vi "Lab2_Light_Filter.vi"() -> ()   [LabVIEW 2022 SP3]
uses:
  <vilib>/DAQmx/read.llb/DAQmx Read (Analog DBL 1Chan 1Samp).vi
  <vilib>/DAQmx/miscellaneous.llb/DAQmx Fill In Error Info.vi
panel:
  in  "stop":bool
  in  "L (0..1)":dbl
  out "error constant":errorcluster
  out "Waveform Chart":cluster{"data":dbl, "y2":dbl}(graph)
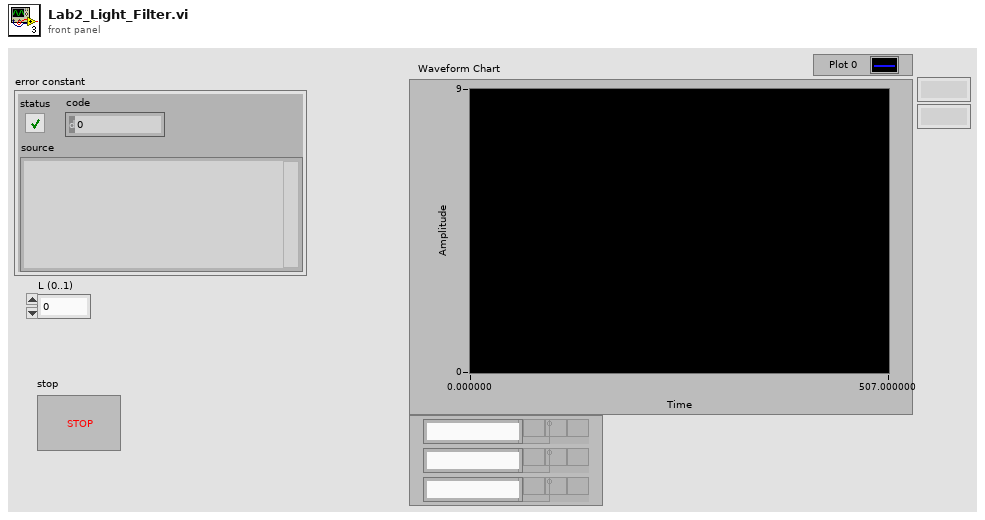
[diagram p1: front panel]
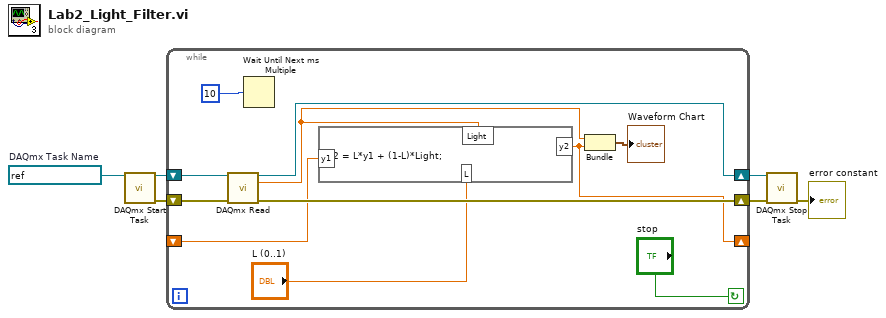
[diagram p0: block diagram]
diagram:
  w2 = refnum<k21> "Light Sensor"  # DAQmx Task Name
  n1 = call <vilib>:"DAQmx Start Task.vi"("task/channels in"=w2) -> ("task out"=w4:refnum<k21>, "error out"=w6:errorcluster)  [unwired: 13 in]
  n2 = while {
    shift-right: [w16] -> w5
    shift-left: w6 -> [w17]
    shift-right: [w14] -> w3
    shift-left: w4 -> [w15]
    shift-right: [w10] -> _
    shift-left: _ -> [w13]
    stop <- "stop" continue-if-true
    n3 = call-poly <vilib>:"DAQmx Read.vi"("task/channels in"=w15, "error in"=w17) -> ("task out"=w14:refnum<k21>, "data"=w11:dbl, "error out"=w16:errorcluster)  [unwired: 11 in]
    n4 = Wait Until Next ms Multiple(millisecond multiple=10) -> ()  [unwired: 1 out]
    n5 = formula code="y2 = L*y1 + (1-L)*Light;"("y1"=w13, "Light"=w11, "L"="L (0..1)") -> ("y2"=w10:dbl)
    n6 = Bundle("data"=w11, "y2"=w10) -> (→"Waveform Chart":cluster{"data":dbl, "y2":dbl})  [unwired: 1 in]
  }
  n7 = call <vilib>:"DAQmx Stop Task.vi"("task/channels in"=w3, "error in"=w5) -> ("error out"=→"error constant":errorcluster)  [unwired: 12 in, 1 out]
